vi "Actor Core.vi"(8 "error in":errorcluster, 11 "CS++SVMonitor in":refnum<class "CS++SVMonitor.lvclass">) -> (0 "error out":errorcluster, 3 "Actor out":refnum<class "Actor.lvclass">)   [LabVIEW 2014, in "CS++SVMonitor.lvlib" / "CS++SVMonitor.lvclass"]
doc: "(<B>Filename</B>: Actor Framework.lvlib:Actor.lvclass:Actor Core.vi)\n\nReceives messages to the actor, reacts to them, and initiates any error handling that may shut the actor down.\n\nDescendant classes may override this VI to append parallel tasks for the actor to complete while it handles messages. Overrides use the Call Parent Method node."
uses:
  CS++SVMonitor.lvclass
  <vilib>/ActorFramework/Actor/Actor.lvclass
  CS++BaseActor/CS++BaseActor.lvclass/CS++BaseActor.ctl
  CS++SVMonitor.lvclass/CS++SVMonitor.ctl
  Classes/CS++ProcessVariables/ProcessVariable/PV.lvclass
  Classes/CS++ProcessVariables/ProcessVariable/PV.lvclass/PV.ctl
  Classes/CS++ProcessVariables/ProcessVariable/Write PV URL.vi
  Classes/CS++ProcessVariables/ProcessVariable/Write Data.vi
  Classes/CS++ProcessVariables/ProcessVariable/Write Timestamp.vi
  Classes/CS++ProcessVariables/ProcessVariable/Write Error.vi
  Classes/CS++ProcessVariables/ProcessVariable/Write Quality.vi
  Classes/CS++ProcessVariables/ProcessVariable/Write status.vi
  CS++PVMonitor/CS++PVMonitor.lvclass
  <vilib>/ActorFramework/Message Enqueuer/Message Enqueuer.lvclass
  CS++PVMonitor Messages/CS++PVUpdate Msg/CS++PVUpdate Msg.lvclass
  CS++BaseActor/CS++BaseActor.lvclass
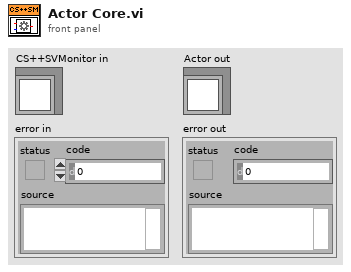
[diagram p1: front panel]
types:
  T1 = cluster{"Stop":refnum<user-event>, "PV Connections":refnum<user-event>}
  T2 = cluster{"Enqueuer":refnum<class "Message Enqueuer.lvclass">, "CS++PVUpdate Msg":refnum<class "CS++PVUpdate Msg.lvclass">}[]
  T3 = cluster{"PV URL":string, "Observers":cluster{"Enqueuer":refnum<class "Message Enqueuer.lvclass">, "CS++PVUpdate Msg":refnum<class "CS++PVUpdate Msg.lvclass">}[]}[]
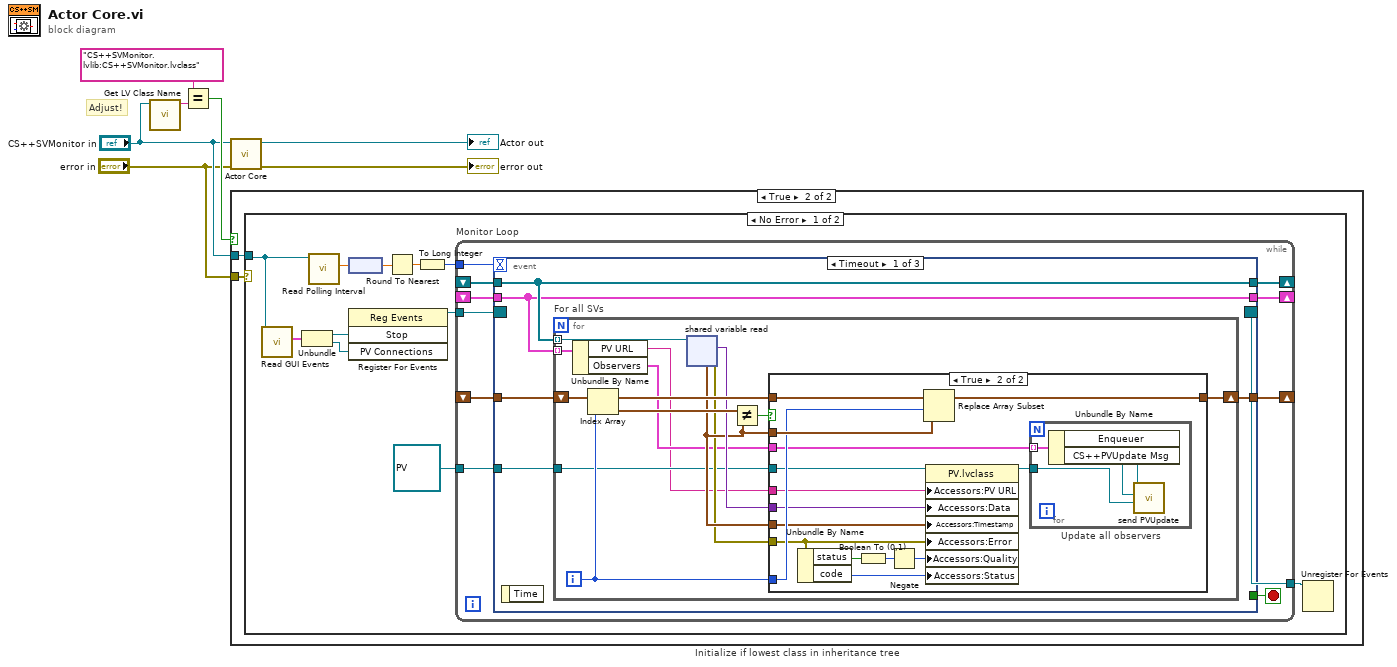
[diagram p0: block diagram]
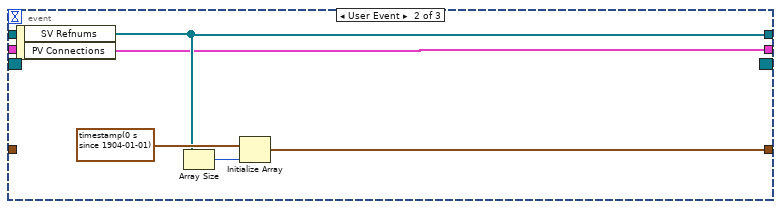
[diagram p4: hidden frame]
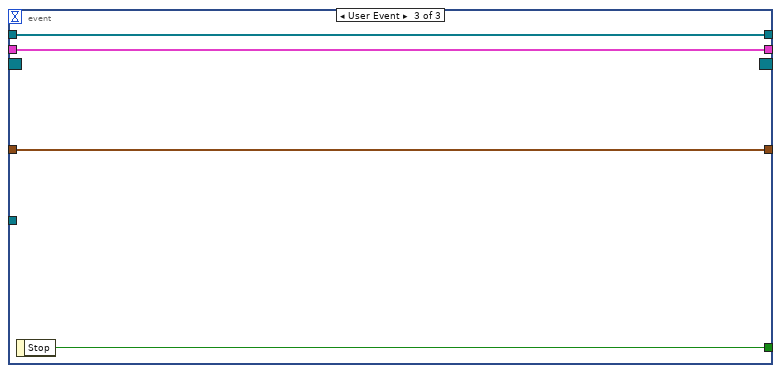
[diagram p5: hidden frame]
diagram:
  # "Adjust!"
  n1 = call <vilib>:"Get LV Class Name.vi"("object"="CS++SVMonitor in") -> ("class name"=w4:string)  [unwired: 9 in, 1 out]
  n2 = Equal?(x="CS++SVMonitor.lvlib:CS++SVMonitor.lvclass" ("class name"), y=w4) -> (x = y?=w3:bool)
  n3 = call-parent "Actor Core.vi"("error in"="error in", "CS++BaseActor in"="CS++SVMonitor in") -> ("error out"=→"error out":errorcluster, "Actor out"=→"Actor out":refnum<class "Actor.lvclass">)  [unwired: 8 in]
  n4 = case "Initialize if lowest class in inheritance tree" shown="True" w3 {
    tunnel: "error in" -> [_ w9]
    tunnel: "CS++SVMonitor in" -> [_ w8]
    frame False {
    }
    frame True {
      n5 = case shown="No Error" w9 {
        tunnel: w8 -> [w14 _]
        frame No Error {
          n6 = call "Read GUI Events.vi"("CS++SVMonitor in"=w14) -> ("GUI Events"=w13:T1)  [unwired: 8 in, 2 out]
          n7 = Unbundle(w13) -> ("Stop"=w12:refnum<user-event>, "PV Connections"=w11:refnum<user-event>)
          n8 = call "Read Polling Interval.vi"("CS++BaseActor in"=w14) -> ("Polling Interval"=w17:dbl[unit])  [unwired: 8 in, 2 out]
          n9 = node(w17) -> (w18:dbl)
          n10 = register-events(w12, w11) -> (reference out=w15:refnum<event-registration>)  [unwired: 2 in, 1 out]
          n11 = Round To Nearest(number=w18) -> (nearest integer value=w19:dbl)
          n12 = To Long Integer(number=w19) -> (32bit integer=w16:i32)
          n13 = while "Monitor Loop" {
            tunnel: w15 -> [w31]
            tunnel: w16 -> [w30]
            tunnel: [w28] -> w10
            shift-right: [w26] -> _
            shift-left: _ -> [w27]
            shift-right: [w24] -> _
            shift-left: _ -> [w25]
            shift-right: [w23] -> _
            shift-left: _ -> [w22]
            tunnel: refnum<class "PV.lvclass"> refnum ("CS++ProcessVariables.lvlib:PV.lvclass") -> [w21]
            stop <- w29 stop-if-true
            n14 = event shown="[0] Timeout" {
              selector: w31 -> [_ _ _]
              dyn-events: [_ _ _] -> w28
              timeout: w30 -> [_ _ _]
              tunnel: [_ _ w78] -> w29
              tunnel: w27 -> [w36 _ w77]
              tunnel: [w35 w71 w77] -> w26
              tunnel: w25 -> [w34 _ w76]
              tunnel: [w34 w72 w76] -> w24
              tunnel: [w32 w70 w75] -> w23
              tunnel: w22 -> [w32 _ w75]
              tunnel: w21 -> [w33 _ _]
              event Timeout {
                n15 = event-data() -> ()  [unwired: 1 in, 1 out]
                n16 = for "For all SVs" {
                  shift-right: [w46] -> w35
                  shift-left: w36 -> [w48]
                  tunnel: w34 -> [w41] mode=indexing
                  tunnel: w32 -> [w40] mode=indexing
                  tunnel: w33 -> [w38]
                  i -> [w47]
                  n17 = Unbundle By Name(w40) -> ("PV URL"=w37:string, "Observers"=w39:T2)
                  n18 = Index Array(array=w48, index=w47) -> (element=w49:timestamp)
                  n19 = shared-variable-read(w41) -> (w42:errorcluster, w44:variant, w43:timestamp)  [unwired: 1 in, 1 out]
                  n20 = Not Equal?(x=w49, y=w43) -> (x != y?=w45:bool)
                  n21 = case shown="True" w45 {
                    tunnel: w43 -> [_ w65]
                    tunnel: w48 -> [w50 w64]
                    tunnel: w47 -> [_ w63]
                    tunnel: [w50 w62] -> w46
                    tunnel: w44 -> [_ w58]
                    tunnel: w43 -> [_ w57]
                    tunnel: w42 -> [_ w56]
                    tunnel: w39 -> [_ w61]
                    tunnel: w38 -> [_ w60]
                    tunnel: w37 -> [_ w51]
                    frame False {
                    }
                    frame True {
                      n22 = Unbundle By Name(w56) -> ("status"=w55:bool, "code"=w52:i32)
                      n23 = Boolean To (0,1)(Boolean=w55) -> (0, 1=w54:i16)
                      n24 = Negate(x=w54) -> (-x=w53:i16)
                      n25 = Replace Array Subset(array=w64, new element=w65, index=w63) -> (w62:timestamp[])
                      n26 = property class="PV.lvclass"(reference=w60, "Accessors:PV URL"=w51, "Accessors:Data"=w58, "Accessors:Timestamp"=w57, "Accessors:Error"=w56, "Accessors:Quality"=w53, "Accessors:Status"=w52) -> (reference out=w59:refnum<class "PV.lvclass">)  [unwired: 1 in, 1 out]
                      n27 = for "Update all observers" {
                        tunnel: w61 -> [w69] mode=indexing
                        tunnel: w59 -> [w66]
                        n28 = Unbundle By Name(w69) -> ("Enqueuer"=w68:refnum<class "Message Enqueuer.lvclass">, "CS++PVUpdate Msg"=w67:refnum<class "CS++PVUpdate Msg.lvclass">)
                        n29 = call "send PVUpdate.vi"("PV"=w66, "CS++PVUpdate Msg in"=w67, "Message Enqueuer in"=w68) -> ()  [unwired: 7 in, 2 out]
                      }
                    }
                  }
                }
              }
              event User Event {
                n30 = event-data() -> ("SV Refnums"=w72:refnum<k21>[], "PV Connections"=w70:T3)  [unwired: 1 in]
                n31 = Array Size(array=w72) -> (size(s)=w74:i32)
                n32 = Initialize Array(timestamp(0 s since 1904-01-01) ("timestamp"), w74) -> (w71:timestamp[])
              }
              event User Event {
                n33 = event-data() -> ("Stop"=w78:bool)  [unwired: 1 in]
              }
            }
          }
          n34 = Unregister For Events(event registration refnum=w10) -> ()  [unwired: 1 in, 1 out]
        }
        frame Error {
        }
      }
    }
  }
